vi "main.vi"(10 "Target":cluster{"Xf":dbl, "Yf":dbl}, 11 "Start Point":cluster{"X0":dbl, "Y0":dbl}) -> (3 "Distance (mm)":dbl)   [LabVIEW 2017]
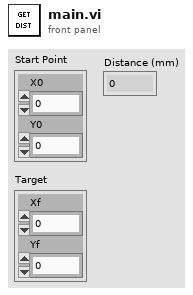
[diagram p1: front panel]
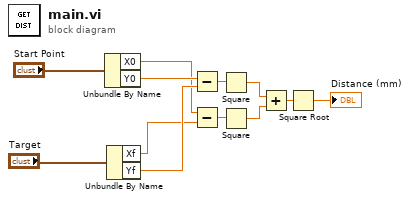
[diagram p0: block diagram]
diagram:
  n1 = Unbundle By Name("Start Point") -> ("X0"=w8:dbl, "Y0"=w10:dbl)
  n2 = Unbundle By Name("Target") -> ("Xf"=w7:dbl, "Yf"=w9:dbl)
  n3 = Subtract(x=w10, y=w9) -> (x-y=w6:dbl)
  n4 = Subtract(x=w8, y=w7) -> (x-y=w5:dbl)
  n5 = Square(x=w6) -> (x^2=w4:dbl)
  n6 = Square(x=w5) -> (x^2=w3:dbl)
  n7 = Add(x=w4, y=w3) -> (x+y=w2:dbl)
  n8 = Square Root(x=w2) -> (sqrt(x)=→"Distance (mm)":dbl)
